vi "String to Connection.vi"(8 "error in":errorcluster, 10 "string":string, 11 "routing and faulting in":T1 format="%.0x") -> (0 "error out":errorcluster, 2 "connection":T2, 3 "routing and faulting out":T1 format="%.0x")   [LabVIEW 2020, in "Routing and Faulting Scripting.lvlib"]
uses:
  Routing and Faulting Scripting.lvlib
  Shared/Connection.ctl
  <vilib>/NI VeriStand/Custom Device API/Custom Device Item Ref.ctl
  <vilib>/regexp/Match Regular Expression.xnode
  Shared/Routing and Faulting Shared.lvlib
  <vilib>/NI VeriStand/Custom Device API/Custom Device API.lvlib
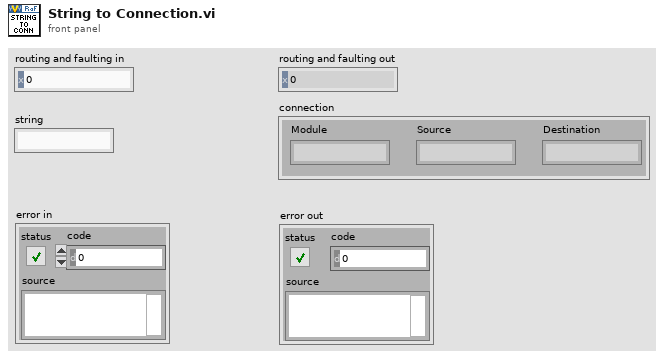
[diagram p1: front panel]
types:
  T1 = typedef "Custom Device API.lvlib/Custom Device Item Ref.ctl" = u64
  T2 = typedef "Routing and Faulting Shared.lvlib/Connection.ctl" = cluster{"Module":string, "Source":string, "Destination":string}
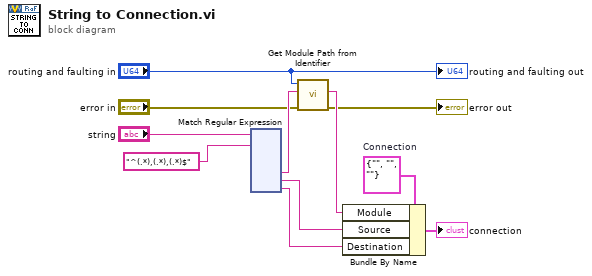
[diagram p0: block diagram]
diagram:
  w9 = T2 {"Module"="", "Source"="", "Destination"=""}  # Connection
  n1 = xnode "Match Regular Expression"("input string"="string", "regular expression"="^(.*),(.*),(.*)$" ("search string")) -> ("submatch 1"=w4:string, "submatch 2"=w7:string, "submatch 3"=w6:string)  [unwired: 4 in, 5 out]
  n2 = call "Get Module Path from Identifier.vi"("error in"="error in", "module identifier"=w4, "routing and faulting in"="routing and faulting in") -> ("error out"=→"error out":errorcluster, "module path"=w5:string)  [unwired: 6 in, 1 out]
  n3 = Bundle By Name(cluster=w9, "Module"=w5, "Source"=w7, "Destination"=w6) -> (→"connection":T2)
  "routing and faulting out" <- "routing and faulting in"
